vi "CalculateDaysSince.vi"() -> ()   [LabVIEW 2018]
panel:
  out "error out":errorcluster
  in  "Date":T1={"day"=1, "month"=enum."May", "year"=2019}
  out "days since date":i32
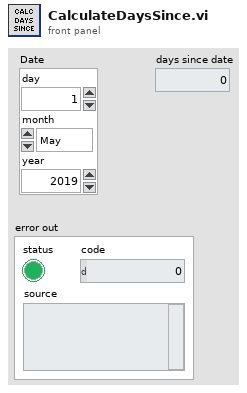
[diagram p1: front panel]
types:
  T1 = cluster{"day":i32, "month":enum16{"Jan", "Feb", "Mar", "Apr", "May", "Jun", "Jul", "Aug", "Sept", "Oct", "Nov", "Dec"}, "year":i32}
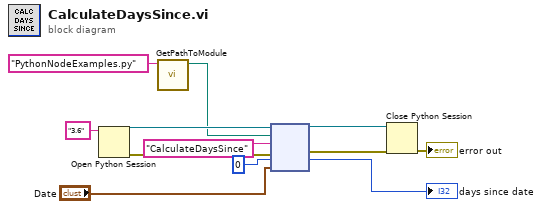
[diagram p0: block diagram]
diagram:
  n1 = Open Python Session(python version="3.6" ("Python version")) -> (session out=w12:refnum<k35>, error out=w5:errorcluster)  [unwired: 2 in]
  n2 = call "GetPathToModule.vi"("module name"="PythonNodeExamples.py") -> ("path to module"=w1:path)  [unwired: 10 in]
  n3 = node(w12, w1, "CalculateDaysSince" ("function name"), w5, 0, "Date") -> (w11:refnum<k35>, w4:errorcluster, →"days since date":i32)  [unwired: 1 in, 2 out]
  n4 = Close Python Session(session in=w11, error in=w4) -> (11:→"error out":errorcluster)
